vi "Get Caraya Namespace.vi"() -> (2 "PPL?":bool, 3 "Namespace":string)   [LabVIEW 2013, in "Caraya.lvlib"]
uses:
  Caraya.lvlib
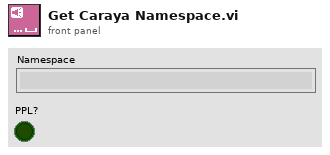
[diagram p1: front panel]
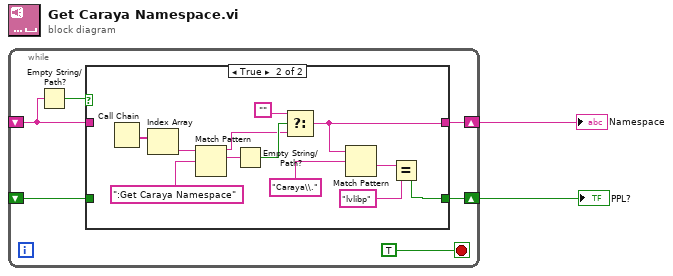
[diagram p0: block diagram]
diagram:
  n1 = while {
    shift-right: [w7] -> w2
    shift-left: _ -> [w6]
    shift-right: [w3] -> w1
    shift-left: _ -> [w4]
    stop <- TRUE stop-if-true
    n2 = Empty String/Path?(string/path=w6) -> (empty?=w8:bool)
    n3 = case shown="True" w8 {
      tunnel: [w10 w15] -> w7
      tunnel: w6 -> [w10 _]
      tunnel: w4 -> [w9 _]
      tunnel: [w9 w11] -> w3
      frame False {
      }
      frame True {
        n4 = Call Chain() -> (call chain=w22:string[])
        n5 = Index Array(array=w22) -> (element=w21:string)  [unwired: 1 in]
        n6 = Match Pattern(string=w21, regular expression=":Get Caraya Namespace") -> (before substring=w16:string, match substring=w19:string)  [unwired: 1 in, 2 out]
        n7 = Empty String/Path?(string/path=w19) -> (empty?=w18:bool)
        n8 = Select(t="", s=w18, f=w16) -> (s? t:f=w15:string)
        n9 = Match Pattern(string=w15, regular expression="Caraya\\.") -> (after substring=w13:string)  [unwired: 1 in, 3 out]
        n10 = Equal?(x=w13, y="lvlibp") -> (x = y?=w11:bool)
      }
    }
  }
  "Namespace" <- w2
  "PPL?" <- w1
